vi "ProgramMicroBlaze_DMA.vi"(7 "Elf File to Download":path=path "C:/Users/kvemishe/Desktop/APAN/mb-DMAboot/mb-DMAboot/xsdk_worspace/helloworld1/Debug/helloworld1.srec", 8 "error in (no error)":errorcluster, 11 "FPGA Interface":refnum<k20>) -> (0 "error out":errorcluster, 2 "DataRecord":T1 {"Address" format="%.0x"; "Data" format="%.0x"}, 3 "FPGA Interface Out":refnum<k20>)   [LabVIEW 2015]
uses:
  BuildELF/DataControl.ctl
  <vilib>/Utility/error.llb/Error Cluster From Error Code.vi
  <vilib>/rvi/errors/niLvFpgaAdjustHostInterfaceError.vi
  <vilib>/rvi/interface/nirviReadWriteControl/nirviReadWriteControl.xnode
  <vilib>/rvi/interface/nirviMethod/nirviMethod.xnode
  NiFpgaLv.dll
  <vilib>/rvi/interface/Simulation/niFpgaSimulationCallBeginRW.vi
  <vilib>/FPGAPlugInAG/Dynamic/niLvFpga_WriteFifo_Dynamic.vi
  <vilib>/rvi/errors/niLvFpgaMergeErrorWithErrorCode.vi
panel:
  out "NumElements":i32
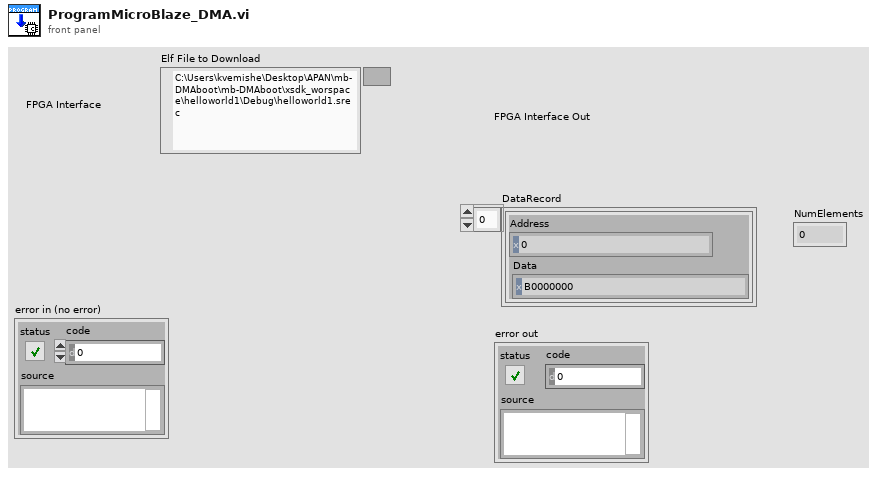
[diagram p1: front panel]
types:
  T1 = typedef "DataControl.ctl" = cluster{"Address":u32, "Data":u32}[]
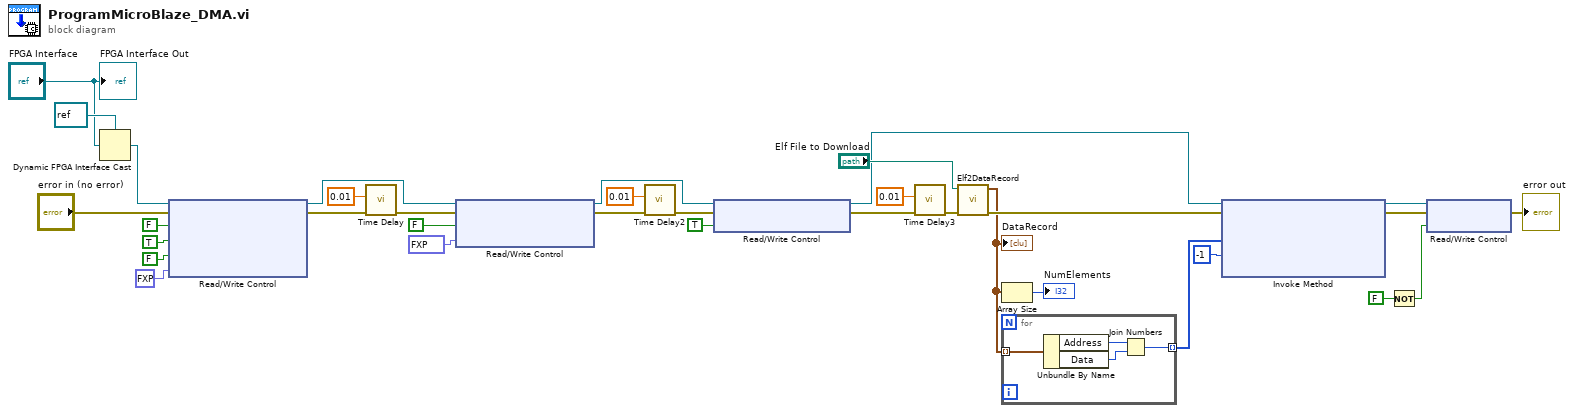
[diagram p0: block diagram]
diagram:
  n1 = Dynamic FPGA Interface Cast(Session In=refnum<k20> refnum ("FPGA Interface"), Type="FPGA Interface") -> (Session Out=w4:refnum<k20>)
  n2 = xnode "Read/Write Control"("FPGA VI Reference In"=w4, "error in"="error in (no error)", "ub1\\reset_rtl"=FALSE ("ub1\\reset_rtl"), "ub1\\BRAM_PORTB_rst"=TRUE ("ub1\\BRAM_PORTB_rst"), "ub1\\BRAM_PORTB_en"=FALSE ("ub1\\BRAM_PORTB_en"), "ub1\\BRAM_PORTB_we"=fxp<+,4,4> 0.0 ("ub1\\BRAM_PORTB_we")) -> ("FPGA VI Reference Out"=w8:refnum<k20>, "error out"=w7:errorcluster)
  n3 = call "Time Delay"("error in (no error)"=w7, "Delay Time (s)"=0.01) -> ("error out"=w9:errorcluster)  [unwired: 9 in]
  n4 = xnode "Read/Write Control"("FPGA VI Reference In"=w8, "error in"=w9, "ub1\\BRAM_PORTB_rst"=FALSE ("ub1\\BRAM_PORTB_en"), "ub1\\BRAM_PORTB_we"=fxp<+,4,4> 15.0 ("ub1\\BRAM_PORTB_we")) -> ("FPGA VI Reference Out"=w11:refnum<k20>, "error out"=w10:errorcluster)
  n5 = call "Time Delay2"("error in (no error)"=w10, "Delay Time (s)"=0.01) -> ("error out"=w12:errorcluster)  [unwired: 9 in]
  n6 = xnode "Read/Write Control"("FPGA VI Reference In"=w11, "error in"=w12, "ub1\\BRAM_PORTB_en"=TRUE ("ub1\\BRAM_PORTB_en")) -> ("FPGA VI Reference Out"=w14:refnum<k20>, "error out"=w13:errorcluster)
  n7 = call "Time Delay3"("error in (no error)"=w13, "Delay Time (s)"=0.01) -> ("error out"=w30:errorcluster)  [unwired: 9 in]
  n8 = call "Elf2DataRecord.vi"("Error In"=w30, "Elf file"="Elf File to Download") -> ("error out"=w31:errorcluster, "DataRecord"=w2:T1)  [unwired: 8 in]
  "DataRecord" <- w2
  n9 = Array Size(array=w2) -> (size(s)=→"NumElements":i32)
  n10 = for {
    tunnel: w2 -> [w38] mode=indexing
    tunnel: [w35] -> w6 mode=indexing
    n11 = Unbundle By Name(w38) -> ("Address"=w37:u32, "Data"=w36:u32)
    n12 = Join Numbers(hi=w37, lo=w36) -> ((hi.lo)=w35:u64)
  }
  n13 = xnode "Invoke Method"("FPGA VI Reference In"=w14, "error in"=w31, "Data"=w6, "Timeout (ms)"=-1) -> ("FPGA VI Reference Out"=w15:refnum<k20>, "error out"=w16:errorcluster)  [unwired: 1 out]
  n14 = Not(x=FALSE) -> (.not. x?=w28:bool)
  n15 = xnode "Read/Write Control"("FPGA VI Reference In"=w15, "error in"=w16, "ub1\\reset_rtl"=w28) -> ("error out"=→"error out":errorcluster)  [unwired: 1 out]
  "FPGA Interface Out" <- "FPGA Interface"
